vi "Get Decimal Separator.vi"() -> (3 "System Decimal separator":string)   [LabVIEW 2013, in "OpenScalar.lvlib"]
uses:
  OpenScalar.lvlib
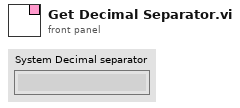
[diagram p1: front panel]
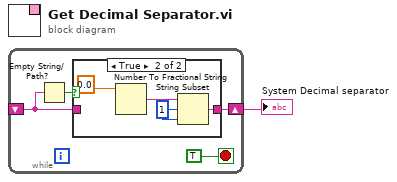
[diagram p0: block diagram]
diagram:
  n1 = while {
    shift-right: [w5] -> w1
    shift-left: _ -> [w2]
    stop <- TRUE stop-if-true
    n2 = Empty String/Path?(string/path=w2) -> (empty?=w3:bool)
    n3 = case shown="True" w3 {
      tunnel: [w6 w7] -> w5
      tunnel: w2 -> [w6 _]
      frame False {
      }
      frame True {
        w8 = 1 ("offset (0)")
        n4 = Number To Fractional String(number=0.0) -> (F-format string=w9:string)  [unwired: 3 in]
        n5 = String Subset(string=w9, offset (0)=w8, length (rest)=w8) -> (substring=w7:string)
      }
    }
  }
  "System Decimal separator" <- w1
